vi "Normaliza_Caracteres.vi"(3 "Trocar por:":string="  ", 4 "Procurar":string="   ", 5 "Entrada":string) -> (1 "Saida":string)   [LabVIEW 2018]
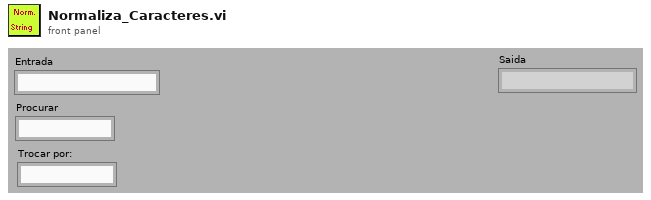
[diagram p1: front panel]
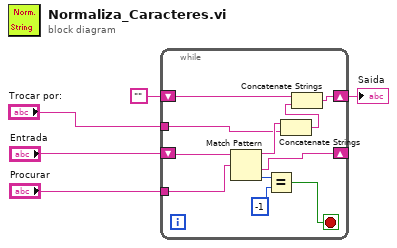
[diagram p0: block diagram]
diagram:
  n1 = while {
    shift-right: [w11] -> w3
    shift-left: "" -> [w10]
    shift-right: [w12] -> _
    shift-left: "Entrada" -> [w13]
    tunnel: "Procurar" -> [w7]
    tunnel: "Trocar por:" -> [w6]
    stop <- w14 stop-if-true
    n2 = Match Pattern(string=w13, regular expression=w7) -> (before substring=w8:string, after substring=w12:string, offset past match=w16:i32)  [unwired: 1 in, 1 out]
    n3 = Equal?(x=w16, y=-1) -> (x = y?=w14:bool)
    n4 = Concatenate Strings(w8, w6) -> (w9:string)
    n5 = Concatenate Strings(w10, w9) -> (w11:string)
  }
  "Saida" <- w3
